vi "SDO_DRIVE_DASH_WRITE.vi"   [LabVIEW 2019]
uses:
  SDO_DRIVE_GLOBALS.vi
  <vilib>/Rock Robotics/Network Tables/NT Write Numeric Array.vi
  <vilib>/Rock Robotics/Network Tables/NT Write Boolean Array.vi
  <vilib>/Rock Robotics/Network Tables/NT Write Boolean.vi
  <vilib>/Rock Robotics/Network Tables/NT Write Number.vi
  <vilib>/Rock Robotics/WPI/ThirdParty/JAS_Junk/TrajLib/Trajectory_Library.lvlib
types:
  T1 = typedef "Trajectory_Library.lvlib/SWERVE_DRIVE_MODULE_STATE.ctl" = cluster{"Speed":dbl, "Angle":T2}
  T2 = typedef "Trajectory_Library.lvlib/ROTATION2D.ctl" = cluster{"VALUE":dbl, "COS":dbl, "SIN":dbl}
  T3 = typedef "Trajectory_Library.lvlib/CHASSIS_SPEEDS.ctl" = cluster{"vX":dbl, "vY":dbl, "vOmega":dbl}
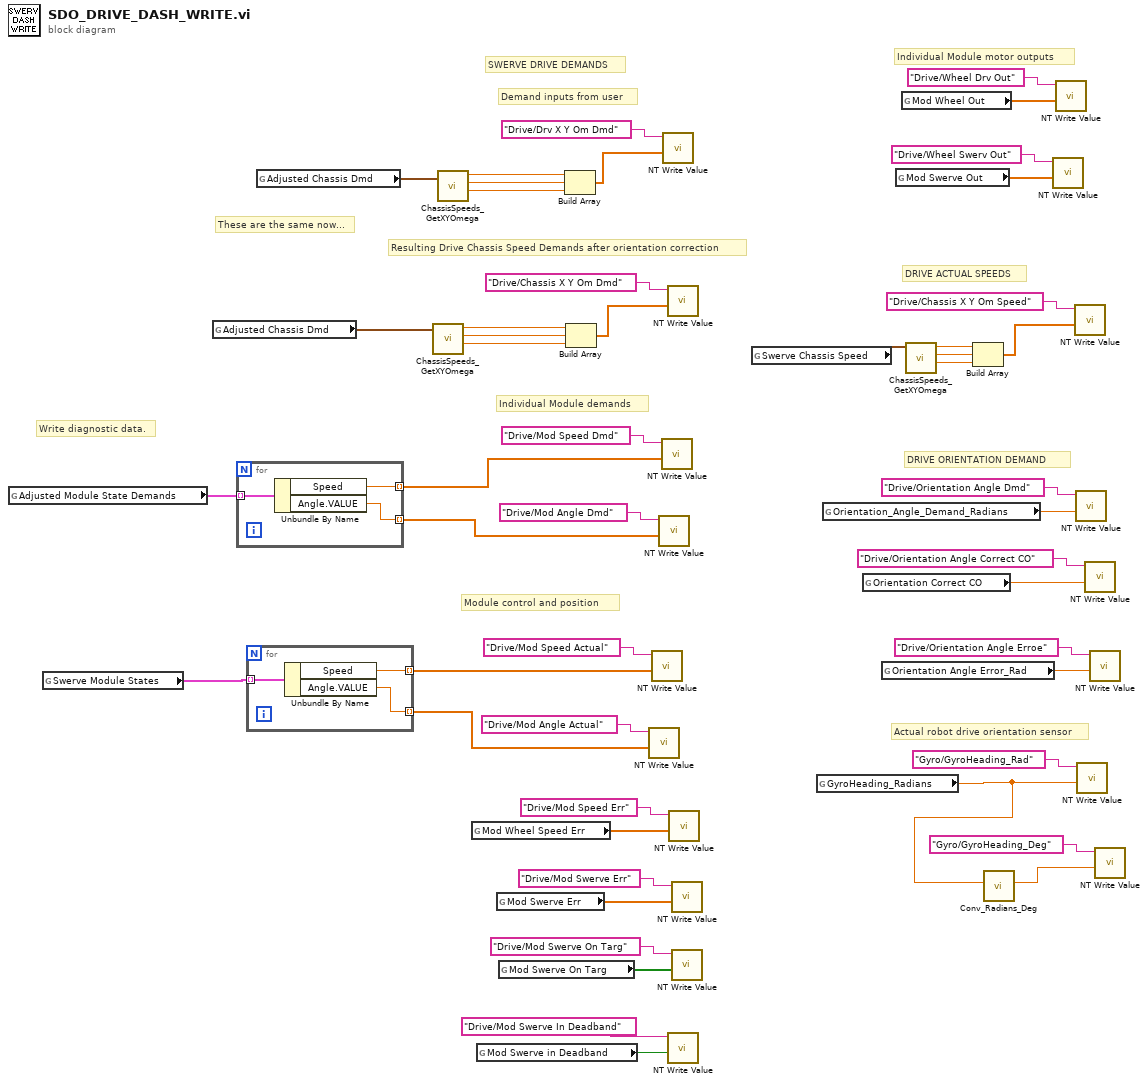
[diagram p0: block diagram]
diagram:
  # "These are the same now..."
  # "Write diagnostic data."
  # "Module control and position"
  # "Actual robot drive orientation sensor"
  # "DRIVE ACTUAL SPEEDS"
  # "DRIVE ORIENTATION DEMAND"
  # "Individual Module motor outputs"
  # "Individual Module demands"
  # "Resulting Drive Chassis Speed Demands after orientation correction"
  # "Demand inputs from user"
  # "SWERVE DRIVE DEMANDS"
  n1 = global read "SDO_DRIVE_GLOBALS.vi" "Adjusted Module State Demands"() -> (w3:T1[])
  n2 = global read "SDO_DRIVE_GLOBALS.vi" "Swerve Module States"() -> (w14:T1[])
  n3 = global read "SDO_DRIVE_GLOBALS.vi" "Adjusted Chassis Dmd"() -> (w11:T3)
  n4 = for {
    tunnel: w3 -> [w53] mode=indexing
    tunnel: [w52] -> w1 mode=indexing
    tunnel: [w51] -> w2 mode=indexing
    n5 = Unbundle By Name(w53) -> ("Speed"=w51:dbl, "Angle.VALUE"=w52:dbl)
  }
  n6 = for {
    tunnel: w14 -> [w56] mode=indexing
    tunnel: [w55] -> w12 mode=indexing
    tunnel: [w54] -> w13 mode=indexing
    n7 = Unbundle By Name(w56) -> ("Speed"=w54:dbl, "Angle.VALUE"=w55:dbl)
  }
  n8 = global read "SDO_DRIVE_GLOBALS.vi" "Adjusted Chassis Dmd"() -> (w18:T3)
  n9 = call <vilib>:"ChassisSpeeds_GetXYOmega.vi"("CHASSIS"=w11) -> ("vAngular"=w8:dbl, "vY"=w9:dbl, "vX"=w10:dbl)  [unwired: 8 in]
  n10 = call <vilib>:"ChassisSpeeds_GetXYOmega.vi"("CHASSIS"=w18) -> ("vAngular"=w15:dbl, "vY"=w16:dbl, "vX"=w17:dbl)  [unwired: 8 in]
  n11 = global read "SDO_DRIVE_GLOBALS.vi" "Mod Wheel Speed Err"() -> (w30:dbl[])
  n12 = global read "SDO_DRIVE_GLOBALS.vi" "Mod Swerve in Deadband"() -> (w28:bool)
  n13 = global read "SDO_DRIVE_GLOBALS.vi" "Mod Swerve Err"() -> (w29:dbl[])
  n14 = global read "SDO_DRIVE_GLOBALS.vi" "Mod Swerve On Targ"() -> (w27:bool[])
  n15 = Build Array(w17, w16, w15) -> (w34:dbl[])
  n16 = Build Array(w10, w9, w8) -> (w36:dbl[])
  n17 = call-poly <vilib>:"NT Write Value.vi"("value"=w12, "name"="Drive/Mod Angle Actual" ("Name")) -> ()  [unwired: 9 in, 1 out]
  n18 = call-poly <vilib>:"NT Write Value.vi"("value"=w13, "name"="Drive/Mod Speed Actual" ("Name")) -> ()  [unwired: 9 in, 1 out]
  n19 = call-poly <vilib>:"NT Write Value.vi"("value"=w1, "name"="Drive/Mod Angle Dmd" ("Name")) -> ()  [unwired: 9 in, 1 out]
  n20 = call-poly <vilib>:"NT Write Value.vi"("value"=w2, "name"="Drive/Mod Speed Dmd" ("Name")) -> ()  [unwired: 9 in, 1 out]
  n21 = call-poly <vilib>:"NT Write Value.vi"("value"=w34, "name"="Drive/Drv X Y Om Dmd" ("Name")) -> ()  [unwired: 9 in, 1 out]
  n22 = call-poly <vilib>:"NT Write Value.vi"("value"=w36, "name"="Drive/Chassis X Y Om Dmd" ("Name")) -> ()  [unwired: 9 in, 1 out]
  n23 = call-poly <vilib>:"NT Write Value.vi"("value"=w28, "name"="Drive/Mod Swerve In Deadband" ("Name")) -> ()  [unwired: 9 in, 1 out]
  n24 = call-poly <vilib>:"NT Write Value.vi"("value"=w30, "name"="Drive/Mod Speed Err" ("Name")) -> ()  [unwired: 9 in, 1 out]
  n25 = call-poly <vilib>:"NT Write Value.vi"("value"=w29, "name"="Drive/Mod Swerve Err" ("Name")) -> ()  [unwired: 9 in, 1 out]
  n26 = call-poly <vilib>:"NT Write Value.vi"("value"=w27, "name"="Drive/Mod Swerve On Targ" ("Name")) -> ()  [unwired: 9 in, 1 out]
  n27 = global read "SDO_DRIVE_GLOBALS.vi" "Swerve Chassis Speed"() -> (w7:T3)
  n28 = global read "SDO_DRIVE_GLOBALS.vi" "GyroHeading_Radians"() -> (w19:dbl)
  n29 = global read "SDO_DRIVE_GLOBALS.vi" "Orientation_Angle_Demand_Radians"() -> (w24:dbl)
  n30 = global read "SDO_DRIVE_GLOBALS.vi" "Orientation Correct CO"() -> (w23:dbl)
  n31 = global read "SDO_DRIVE_GLOBALS.vi" "Orientation Angle Error_Rad"() -> (w22:dbl)
  n32 = global read "SDO_DRIVE_GLOBALS.vi" "Mod Swerve Out"() -> (w26:dbl[])
  n33 = global read "SDO_DRIVE_GLOBALS.vi" "Mod Wheel Out"() -> (w25:dbl[])
  n34 = call <vilib>:"ChassisSpeeds_GetXYOmega.vi"("CHASSIS"=w7) -> ("vAngular"=w4:dbl, "vY"=w5:dbl, "vX"=w6:dbl)  [unwired: 8 in]
  n35 = Build Array(w6, w5, w4) -> (w44:dbl[])
  n36 = call <vilib>:"Conv_Radians_Deg.vi"("Radians"=w19) -> ("Degrees"=w20:dbl)  [unwired: 10 in]
  n37 = call-poly <vilib>:"NT Write Value.vi"("value"=w26, "name"="Drive/Wheel Swerv Out" ("Name")) -> ()  [unwired: 9 in, 1 out]
  n38 = call-poly <vilib>:"NT Write Value.vi"("value"=w25, "name"="Drive/Wheel Drv Out" ("Name")) -> ()  [unwired: 9 in, 1 out]
  n39 = call-poly <vilib>:"NT Write Value.vi"("value"=w44, "name"="Drive/Chassis X Y Om Speed" ("Name")) -> ()  [unwired: 9 in, 1 out]
  n40 = call-poly <vilib>:"NT Write Value.vi"("value"=w24, "name"="Drive/Orientation Angle Dmd" ("Name")) -> ()  [unwired: 9 in, 1 out]
  n41 = call-poly <vilib>:"NT Write Value.vi"("value"=w19, "name"="Gyro/GyroHeading_Rad" ("Name")) -> ()  [unwired: 9 in, 1 out]
  n42 = call-poly <vilib>:"NT Write Value.vi"("value"=w23, "name"="Drive/Orientation Angle Correct CO" ("Name")) -> ()  [unwired: 9 in, 1 out]
  n43 = call-poly <vilib>:"NT Write Value.vi"("value"=w22, "name"="Drive/Orientation Angle Erroe" ("Name")) -> ()  [unwired: 9 in, 1 out]
  n44 = call-poly <vilib>:"NT Write Value.vi"("value"=w20, "name"="Gyro/GyroHeading_Deg" ("Name")) -> ()  [unwired: 9 in, 1 out]
